vi "Set FPGA constants.vi"(8 "error in (no error)":errorcluster, 11 "AODAcq in":refnum<class "AODAcq.lvclass">) -> (0 "error out":errorcluster, 3 "AODAcq out":refnum<class "AODAcq.lvclass">)   [LabVIEW 2011, in "AODAcq.lvclass"]
uses:
  AODAcq.lvclass
  FPGA_Control/AODCalibration.ctl
  <vilib>/Utility/error.llb/Error Cluster From Error Code.vi
  Program Files/National Instruments/LabVIEW 2011/Targets/NI/FPGA/StockFPGA_IntfPrivate/ScriptTemplates/StockFPGA_PlugInRead32.vi
  <vilib>/rvi/errors/niLvFpgaAdjustHostInterfaceError.vi
  <vilib>/rvi/interface/nirviReadWriteControl/nirviReadWriteControl.xnode
  FPGA_Control/AODRef.ctl
  FPGA_Control/FPGA Bitfiles/AODControl_FPGATarget_5751Acquire_F1CF9257.lvbitx
  FPGA_Control/AOD Control (FPGA).vi
  NiFpgaLv.dll
  <vilib>/FPGAPlugInAG/PXIe-7965R/niLvFpga_Read32_PXIe-7965R.vi
  <vilib>/rvi/interface/nirviReadWriteControl/niFpgaRWControlAccessTimeoutTemplate.vi
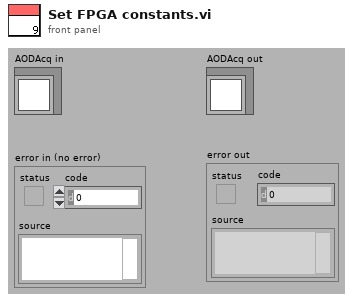
[diagram p1: front panel]
types:
  T1 = typedef "AODCalibration.ctl" = cluster{"XHP ChirpGain":fxp<+/-,16,2>, "YHP ChirpGain":fxp<+/-,16,2>, "XLP ChirpGain":fxp<+/-,16,2>, "YLP ChirpGain":fxp<+/-,16,2>}
  T2 = typedef "AODRef.ctl" = refnum<k20>
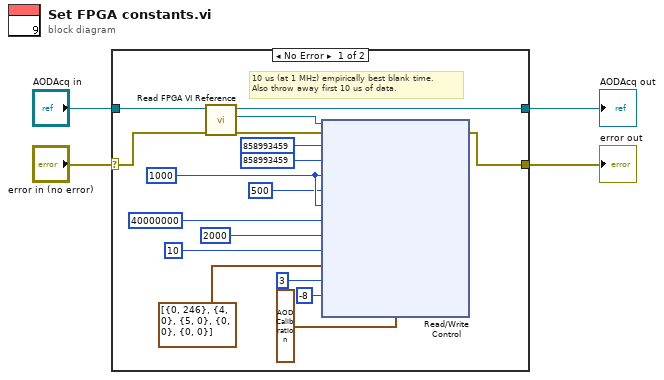
[diagram p0: block diagram]
diagram:
  n1 = case shown="No Error" "error in (no error)" {
    selector: "error in (no error)" -> [w13 w23]
    tunnel: [w12 w23] -> w3
    tunnel: [w20 w22] -> w1
    tunnel: "AODAcq in" -> [w21 w22]
    frame No Error {
      w8 = u32 1000 ("Downsample")
      # "10 us (at 1 MHz) empirically best blank time.\nAlso throw away first 10 us of data."
      n2 = call-dynamic "Read FPGA VI Reference.vi"("error in (no error)"=w13, "AODAcq in"=w21) -> ("error out"=w18:errorcluster, "FPGA VI Reference"=w19:T2, "AODAcq out"=w20:refnum<class "AODAcq.lvclass">)  [unwired: 7 in]
      n3 = xnode "Read/Write Control"("FPGA VI Reference In"=w19, "error in"=w18, "AOD.HP Center Frequency"=u32 858993459 ("LP Center Frequency"), "AOD.LP Center Frequency"=u32 858993459 ("LP Center Frequency"), "Setup.Downsample"=w8, "AOD.BlankSamples"=u16 500, "AOD.ThrowawaySamples"=w8, "Update IO timeout"=u32 40000000 ("Setup.PMT Timeout"), "AOD.UpdatesPerPoint"=u32 2000, "Comm.P high"=u32 10 ("P high"), "Debug.FinishedSetting"=cluster{"Address":u8, "Value":u32}[] [{"Address"=0, "Value"=246}, {"Address"=4, "Value"=0}, {"Address"=5, "Value"=0}, {"Address"=0, "Value"=0}, {"Address"=0, "Value"=0}], "Debug.FinishedSettingSize"=i16 3, "Setup.BitShift"=i16 -8, "AOD.Calibration"=T1 {"XHP ChirpGain"=1.0, "YHP ChirpGain"=1.0, "XLP ChirpGain"=1.0, "YLP ChirpGain"=1.0}) -> ("error out"=w12:errorcluster)  [unwired: 1 out]
    }
    frame Error {
    }
  }
  "error out" <- w3
  "AODAcq out" <- w1
